vi "Read Currently Temperature.vi"(8 "error in (no error)":errorcluster, 11 "Simulated_Cooler in":refnum<class "Simulated_Cooler.lvclass">) -> (0 "error out":errorcluster, 2 "Currently Temperature":i16, 3 "Simulated_Cooler out":refnum<class "Simulated_Cooler.lvclass">)   [LabVIEW 2018, in "Simulated_Cooler.lvclass"]
uses:
  Simulated_Cooler.lvclass
  Simulated_Cooler.lvclass/Simulated_Cooler.ctl
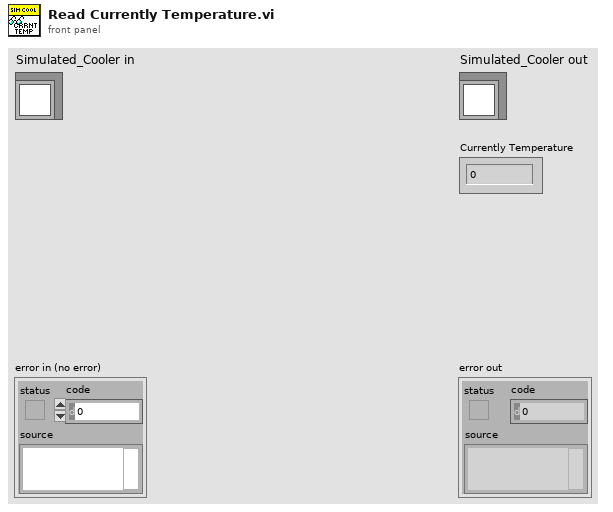
[diagram p1: front panel]
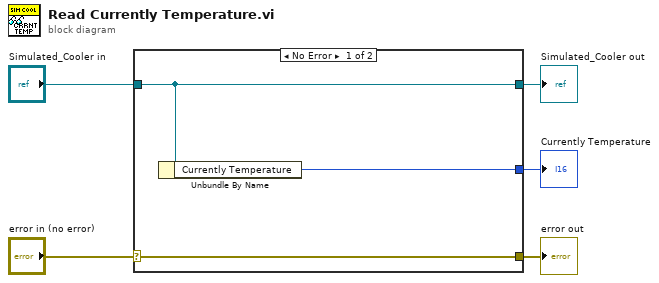
[diagram p0: block diagram]
diagram:
  n1 = case shown="No Error" "error in (no error)" {
    selector: "error in (no error)" -> [w8 w9]
    tunnel: [w8 w9] -> w4
    tunnel: [w7 w10] -> w2
    tunnel: "Simulated_Cooler in" -> [w7 w10]
    tunnel: [w6 _] -> w1
    frame No Error {
      n2 = Unbundle By Name(w7) -> ("Currently Temperature"=w6:i16)
    }
    frame Error {
    }
  }
  "error out" <- w4
  "Simulated_Cooler out" <- w2
  "Currently Temperature" <- w1
